vi "TriggerbasedProgramm2.vi"() -> ()   [LabVIEW 2024]
uses:
  <vilib>/DAQmx/read.llb/DAQmx Read (Analog 1D Wfm NChan NSamp).vi
  <vilib>/DAQmx/create/channels.llb/DAQmx Create Channel (AI-Voltage-Basic).vi
  <vilib>/DAQmx/configure/timing.llb/DAQmx Timing (Sample Clock).vi
  <vilib>/DAQmx/miscellaneous.llb/DAQmx Fill In Error Info.vi
panel:
  in  "File Name 2":string
  in  "Folder to save file to 2":path=path "A:/Source Localization/Material Evaluation paper/Dataset/Microphone Characterization/Clean Source"
  in  "physical channels 2":tag="cDAQ2Mod1/ai0, cDAQ2Mod1/ai3"
  in  "Stop Visualization":bool
  out "?":dynamicdata(graph)=[{"t0"=timestamp(3806599236.6321588 s since 1904-01-01), "dt"=4.999999999999579e-07, "Y"=array[202167 elements], "attributes"=variant("NI_ChannelName"=variant(string "cDAQ2Mod1/ai0"), "NI_UnitDescription"=variant(string "Volts"))}]
  out "?":dynamicdata(graph)=[{"t0"=timestamp(3806599236.6321588 s since 1904-01-01), "dt"=4.999999999999579e-07, "Y"=array[202167 elements], "attributes"=variant("NI_ChannelName"=variant(string "cDAQ2Mod1/ai1"), "NI_UnitDescription"=variant(string "Volts"))}]
  in  "File Logging":bool
  in  "Stop Acquisition":bool
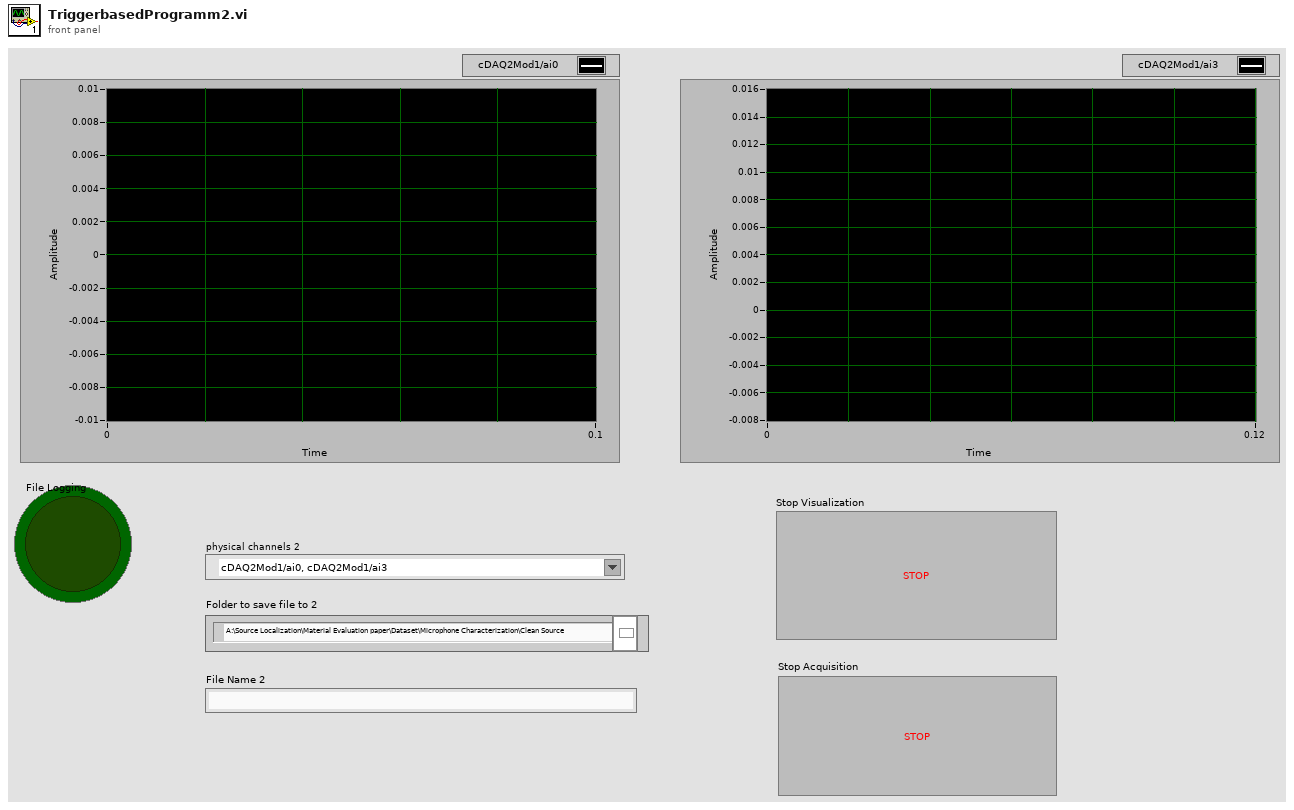
[diagram p1: front panel]
types:
  T1 = enum16{"open", "open or create", "create or replace", "create", "open (read-only)"}
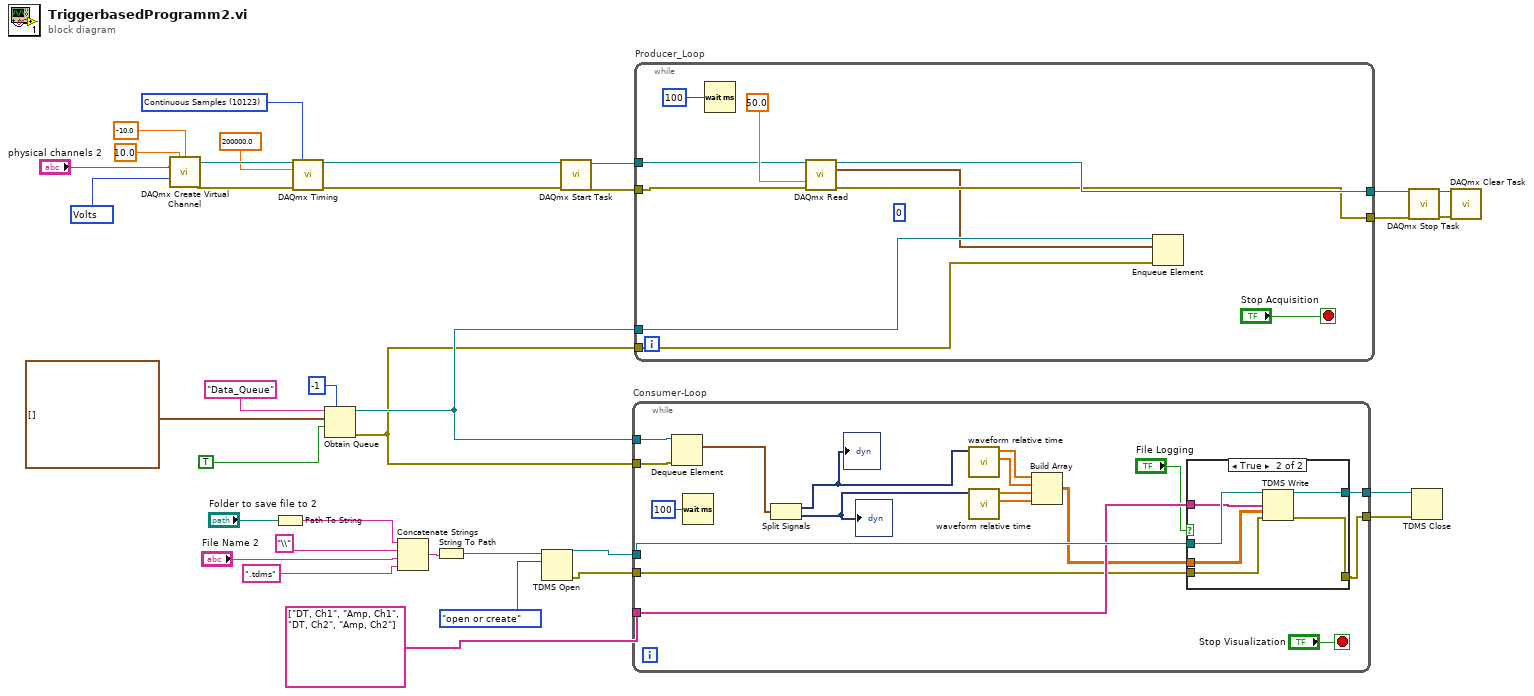
[diagram p0: block diagram]
diagram:
  w7 = 10123 items=["Finite Samples"=10178, "Continuous Samples"=10123, "Hardware Timed Single Point"=12522] ("sample mode")
  w13 = 10348 items=["Volts"=10348, "From Custom Scale"=10065] ("units")
  n1 = call-poly <vilib>:"DAQmx Create Virtual Channel.vi"("maximum value"=10.0, "minimum value"=-10.0, "physical channels"="physical channels 2", "units"=w13) -> ("task out"=w9:refnum<k21>, "error out"=w8:errorcluster)  [unwired: 10 in]
  n2 = Path To String(path="Folder to save file to 2") -> (string=w32:string)
  n3 = call-poly <vilib>:"DAQmx Timing.vi"("task/channels in"=w9, "sample mode"=w7, "rate"=200000.0, "error in"=w8) -> ("task out"=w1:refnum<k21>, "error out"=w2:errorcluster)  [unwired: 10 in]
  n4 = Obtain Queue(max queue size (-1, unlimited)=-1, name (unnamed)="Data_Queue", element data type=waveform(dbl)[] [], create if not found? (T)=TRUE) -> (queue out=w22:refnum<queue>, error out=w17:errorcluster)  [unwired: 1 in, 1 out]
  n5 = Concatenate Strings(w32, "\\" ("string"), "File Name 2", ".tdms" ("string")) -> (w31:string)
  n6 = String To Path(string=w31) -> (path=w28:path)
  n7 = TDMS Open(10:T1."open or create" ("operation (0:open)"), 11:w28) -> (0:w20:errorcluster, 3:w21:refnum<k34>)  [unwired: 5 in]
  n8 = call <vilib>:"DAQmx Start Task.vi"("task/channels in"=w1, "error in"=w2) -> ("task out"=w5:refnum<k21>, "error out"=w6:errorcluster)  [unwired: 12 in]
  n9 = while "Consumer-Loop" {
    tunnel: w22 -> [w53]
    tunnel: w21 -> [w51]
    tunnel: w20 -> [w41]
    tunnel: w17 -> [w52]
    tunnel: string[] ["DT, Ch1", "Amp, Ch1", "DT, Ch2", "Amp, Ch2"] ("channel name(s) in (Untitled)") -> [w50]
    tunnel: [w43] -> w15
    tunnel: [w40] -> w12
    stop <- "Stop Visualization" stop-if-true
    n10 = Dequeue Element(queue=w53, error in (no error)=w52) -> (element=w36:waveform(dbl)[])  [unwired: 1 in, 3 out]
    n11 = Wait (ms)(milliseconds to wait=u32 100) -> ()  [unwired: 1 out]
    n12 = Split Signals(w36) -> (w42:dynamicdata, w45:dynamicdata)  [unwired: 2 in]
    "?" <- w42
    "?" <- w45
    n13 = call "waveform relative time.vi"("signal in"=w42) -> ("Y"=w46:dbl[], "Relative Time"=w47:dbl[])  [unwired: 7 in, 2 out]
    n14 = call "waveform relative time.vi"("signal in"=w45) -> ("Y"=w49:dbl[], "Relative Time"=w48:dbl[])  [unwired: 7 in, 2 out]
    n15 = Build Array(w47, w46, w48, w49) -> (w44:dbl[][])
    n16 = case shown="True" "File Logging" {
      tunnel: w51 -> [w54 w61]
      tunnel: w50 -> [_ w60]
      tunnel: w44 -> [_ w59]
      tunnel: [w54 w58] -> w43
      tunnel: w41 -> [w55 w57]
      tunnel: [w55 w56] -> w40
      frame False {
      }
      frame True {
        n17 = TDMS Write(0:w61, 7:w60, 9:w59, 11:w57) -> (4:w58:refnum<k34>, 15:w56:errorcluster)  [unwired: 2 in, 2 out]
      }
    }
  }
  n18 = while "Producer_Loop" {
    tunnel: w22 -> [w71]
    tunnel: w17 -> [w70]
    tunnel: [w69] -> w19
    tunnel: [w68] -> w18
    tunnel: w5 -> [w64]
    tunnel: w6 -> [w63]
    stop <- "Stop Acquisition" stop-if-true
    (unwired) 0 ("index")
    n19 = Wait (ms)(milliseconds to wait=u32 100) -> ()  [unwired: 1 out]
    n20 = call-poly <vilib>:"DAQmx Read.vi"("task/channels in"=w64, "timeout"=50.0, "error in"=w63) -> ("task out"=w69:refnum<k21>, "data"=w62:waveform(dbl)[], "error out"=w68:errorcluster)  [unwired: 10 in]
    n21 = Enqueue Element(queue=w71, element=w62, error in (no error)=w70) -> ()  [unwired: 1 in, 3 out]
  }
  n22 = call <vilib>:"DAQmx Stop Task.vi"("task/channels in"=w19, "error in"=w18) -> ("task out"=w27:refnum<k21>, "error out"=w26:errorcluster)  [unwired: 12 in]
  n23 = TDMS Close(8:w12, 11:w15) -> ()  [unwired: 2 out]
  n24 = call <vilib>:"DAQmx Clear Task.vi"("task in"=w27, "error in"=w26) -> ()  [unwired: 13 in, 1 out]
